vi "HandleObservationSync.vi"(8 "error in (no error)":errorcluster, 11 "S4GUI in":refnum<class "S4GUI.lvclass">) -> (0 "error out":errorcluster, 3 "S4GUI out":refnum<class "S4GUI.lvclass">)   [LabVIEW 2018, in "S4GUI.lvclass"] (continued)
          n221 = call "Read Instrument.lvclass.vi"("error in (no error)"=w570, "S4ACS_GUI in"=w571) -> ("error out"=w541:errorcluster, "Instrument.lvclass"=w542:refnum<class "Instrument.lvclass">, "S4ACS_GUI out"=w572:refnum<class "S4GUI.lvclass">)  [unwired: 7 in]
          n222 = disable-structure shown="Enabled" {
            disable-tunnel: w542 -> [w576 w589]
            disable-tunnel: w541 -> [w575 w588]
            disable-tunnel: [w574 w589] -> w540
            disable-tunnel: [w573 w588] -> w539
            frame Disabled {
              n223 = call "Read WPROT.vi"("error in (no error)"=w575, "Instrument in"=w576) -> ("error out"=w579:errorcluster, "Opt_Selector.lvclass"=w580:refnum<class "Opt_Selector.lvclass">, "Instrument out"=w586:refnum<class "Instrument.lvclass">)  [unwired: 7 in]
              n224 = call-dynamic "Read State Machine.vi"("error in (no error)"=w579, "Device in"=w580) -> ("error out"=w582:errorcluster, "State Machine.lvclass"=w584:refnum<class "State Machine.lvclass">, "Device out"=w581:refnum<class "Opt_Selector.lvclass">)  [unwired: 7 in]
              n225 = call "Next State.vi"("error in (no error)"=w582, "New_State"=30, "State Machine in"=w584) -> ("error out"=w578:errorcluster, "State Machine out"=w577:refnum<class "State Machine.lvclass">)  [unwired: 7 in]
              n226 = call-dynamic "Write State Machine.vi"("error in (no error)"=w578, "State Machine.lvclass"=w577, "Device in"=w581) -> ("error out"=w585:errorcluster, "Device out"=w587:refnum<class "Opt_Selector.lvclass">)  [unwired: 7 in]
              n227 = call "Write WPROT.vi"("error in (no error)"=w585, "Opt_Selector.lvclass"=w587, "Instrument in"=w586) -> ("error out"=w573:errorcluster, "Instrument out"=w574:refnum<class "Instrument.lvclass">)  [unwired: 7 in]
            }
            frame Enabled {
              # "depois do homing no WPSEL, o homing do WPROT é feito automaticamente pelo ICS"
            }
          }
          n228 = call "Read ASEL.vi"("error in (no error)"=w539, "Instrument in"=w540) -> ("error out"=w556:errorcluster, "Opt_Selector.lvclass"=w557:refnum<class "Opt_Selector.lvclass">, "Instrument out"=w563:refnum<class "Instrument.lvclass">)  [unwired: 7 in]
          n229 = call-dynamic "Read State Machine.vi"("error in (no error)"=w556, "Device in"=w557) -> ("error out"=w559:errorcluster, "State Machine.lvclass"=w561:refnum<class "State Machine.lvclass">, "Device out"=w558:refnum<class "Opt_Selector.lvclass">)  [unwired: 7 in]
          n230 = call "Next State.vi"("error in (no error)"=w559, "New_State"=30, "State Machine in"=w561) -> ("error out"=w555:errorcluster, "State Machine out"=w554:refnum<class "State Machine.lvclass">)  [unwired: 7 in]
          n231 = call-dynamic "Write State Machine.vi"("error in (no error)"=w555, "State Machine.lvclass"=w554, "Device in"=w558) -> ("error out"=w562:errorcluster, "Device out"=w564:refnum<class "Opt_Selector.lvclass">)  [unwired: 7 in]
          n232 = Increment(x=w565) -> (x+1=w567:u32)
          n233 = call "Write ASEL.vi"("error in (no error)"=w562, "Opt_Selector.lvclass"=w564, "Instrument in"=w563) -> ("error out"=w537:errorcluster, "Instrument out"=w538:refnum<class "Instrument.lvclass">)  [unwired: 7 in]
          n234 = call "Read GMIR.vi"("error in (no error)"=w537, "Instrument in"=w538) -> ("error out"=w545:errorcluster, "Opt_Continuous.lvclass"=w546:refnum<class "Opt_Continuous.lvclass">, "Instrument out"=w552:refnum<class "Instrument.lvclass">)  [unwired: 7 in]
          n235 = call-dynamic "Read State Machine.vi"("error in (no error)"=w545, "Device in"=w546) -> ("error out"=w548:errorcluster, "State Machine.lvclass"=w550:refnum<class "State Machine.lvclass">, "Device out"=w547:refnum<class "Opt_Continuous.lvclass">)  [unwired: 7 in]
          n236 = call "Next State.vi"("error in (no error)"=w548, "New_State"=30, "State Machine in"=w550) -> ("error out"=w544:errorcluster, "State Machine out"=w543:refnum<class "State Machine.lvclass">)  [unwired: 7 in]
          n237 = call-dynamic "Write State Machine.vi"("error in (no error)"=w544, "State Machine.lvclass"=w543, "Device in"=w547) -> ("error out"=w551:errorcluster, "Device out"=w553:refnum<class "Opt_Continuous.lvclass">)  [unwired: 7 in]
          n238 = call "Write GMIR.vi"("error in (no error)"=w551, "Opt_Continuous.lvclass"=w553, "Instrument in"=w552) -> ("error out"=w536:errorcluster, "Instrument out"=w535:refnum<class "Instrument.lvclass">)  [unwired: 7 in]
          n239 = call "Write Instrument.lvclass.vi"("error in (no error)"=w536, "Instrument.lvclass"=w535, "S4ACS_GUI in"=w572) -> ("error out"=w569:errorcluster, "S4ACS_GUI out"=w568:refnum<class "S4GUI.lvclass">)  [unwired: 7 in]
          n240 = Bundle By Name(cluster=w568, "Obs_state"=w567) -> (w566:refnum<class "S4GUI.lvclass">)
        }
        frame 223 {
          # "Espera terminar o homing de WPROT,ASEL e GFOC\nantes de seguir para o próximo estado."
          n241 = call "Read Instrument.lvclass.vi"("error in (no error)"=w614, "S4ACS_GUI in"=w615) -> ("error out"=w600:errorcluster, "Instrument.lvclass"=w601:refnum<class "Instrument.lvclass">, "S4ACS_GUI out"=w609:refnum<class "S4GUI.lvclass">)  [unwired: 7 in]
          n242 = call "Read ASEL.vi"("error in (no error)"=w600, "Instrument in"=w601) -> ("error out"=w605:errorcluster, "Opt_Selector.lvclass"=w591:refnum<class "Opt_Selector.lvclass">)  [unwired: 7 in, 1 out]
          n243 = call "Read GMIR.vi"("error in (no error)"=w600, "Instrument in"=w601) -> ("error out"=w602:errorcluster, "Opt_Continuous.lvclass"=w590:refnum<class "Opt_Continuous.lvclass">)  [unwired: 7 in, 1 out]
          n244 = disable-structure shown="Enabled" {
            disable-tunnel: [w619 w625] -> w608
            disable-tunnel: w601 -> [w618 _]
            disable-tunnel: w600 -> [w617 w625]
            disable-tunnel: [w616 0 ("State")] -> w599
            frame Disabled {
              n245 = call "Read WPROT.vi"("error in (no error)"=w617, "Instrument in"=w618) -> ("error out"=w621:errorcluster, "Opt_Selector.lvclass"=w620:refnum<class "Opt_Selector.lvclass">)  [unwired: 7 in, 1 out]
              n246 = call-dynamic "Read State Machine.vi"("error in (no error)"=w621, "Device in"=w620) -> ("error out"=w622:errorcluster, "State Machine.lvclass"=w623:refnum<class "State Machine.lvclass">)  [unwired: 7 in, 1 out]
              n247 = call-dynamic "Read State.vi"("error in (no error)"=w622, "State Machine in"=w623) -> ("error out"=w619:errorcluster, "State"=w616:i32)  [unwired: 7 in, 1 out]
            }
            frame Enabled {
            }
          }
          n248 = call-dynamic "Read State Machine.vi"("error in (no error)"=w605, "Device in"=w591) -> ("error out"=w606:errorcluster, "State Machine.lvclass"=w607:refnum<class "State Machine.lvclass">)  [unwired: 7 in, 1 out]
          n249 = call-dynamic "Read State Machine.vi"("error in (no error)"=w602, "Device in"=w590) -> ("error out"=w603:errorcluster, "State Machine.lvclass"=w604:refnum<class "State Machine.lvclass">)  [unwired: 7 in, 1 out]
          n250 = Increment(x=w611) -> (x+1=w610:u32)
          n251 = call-dynamic "Read State.vi"("error in (no error)"=w606, "State Machine in"=w607) -> ("error out"=w594:errorcluster, "State"=w598:i32)  [unwired: 7 in, 1 out]
          n252 = call-dynamic "Read State.vi"("error in (no error)"=w603, "State Machine in"=w604) -> ("error out"=w593:errorcluster, "State"=w597:i32)  [unwired: 7 in, 1 out]
          n253 = Compound Arithmetic op=ADD(w599, w598, w597) -> (w596:i32)
          n254 = Equal To 0?(x=w596) -> (x = 0?=w595:bool)
          n255 = Merge Errors(w608, w594, w593) -> (w592:errorcluster)
          n256 = Select(t=w610, s=w595, f=w611) -> (s? t:f=w612:u32)
          n257 = Bundle By Name(cluster=w609, "Obs_state"=w612) -> (w613:refnum<class "S4GUI.lvclass">)
        }
        frame 224 {
          # "40 x 0.25 = 10s"
          # "40 x 0.25 = 10s"
          # "40 x 0.25 = 10s"
          # "Manda WPSEL para OFF, CALW para OFF e ASEL para OFF"
          n258 = call "Read Instrument.lvclass.vi"("error in (no error)"=w699, "S4ACS_GUI in"=w700) -> ("error out"=w685:errorcluster, "Instrument.lvclass"=w686:refnum<class "Instrument.lvclass">, "S4ACS_GUI out"=w701:refnum<class "S4GUI.lvclass">)  [unwired: 7 in]
          n259 = call "Read WPSEL.vi"("error in (no error)"=w685, "Instrument in"=w686) -> ("error out"=w681:errorcluster, "Opt_Selector.lvclass"=w680:refnum<class "Opt_Selector.lvclass">, "Instrument out"=w693:refnum<class "Instrument.lvclass">)  [unwired: 7 in]
          n260 = call "Write target.vi"("error in (no error)"=w681, "target"=80.0, "Optics in"=w680) -> ("error out"=w684:errorcluster, "Optics out"=w679:refnum<class "Opt_Selector.lvclass">)  [unwired: 7 in]
          n261 = call "Write target name.vi"("error in (no error)"=w684, "target name"="OFF", "Optics in"=w679) -> ("error out"=w677:errorcluster, "Optics out"=w678:refnum<class "Opt_Selector.lvclass">)  [unwired: 7 in]
          n262 = call-dynamic "Read State Machine.vi"("error in (no error)"=w677, "Device in"=w678) -> ("error out"=w688:errorcluster, "State Machine.lvclass"=w690:refnum<class "State Machine.lvclass">, "Device out"=w687:refnum<class "Opt_Selector.lvclass">)  [unwired: 7 in]
          n263 = call "Next State.vi"("error in (no error)"=w688, "New_State"=1, "State Machine in"=w690) -> ("error out"=w638:errorcluster, "State Machine out"=w640:refnum<class "State Machine.lvclass">)  [unwired: 7 in]
          n264 = call-dynamic "Write Timer.vi"("error in (no error)"=w638, "Timer"=u32 40, "State Machine in"=w640) -> ("error out"=w637:errorcluster, "State Machine out"=w639:refnum<class "State Machine.lvclass">)  [unwired: 7 in]
          n265 = call-dynamic "Write State Machine.vi"("error in (no error)"=w637, "State Machine.lvclass"=w639, "Device in"=w687) -> ("error out"=w692:errorcluster, "Device out"=w694:refnum<class "Opt_Selector.lvclass">)  [unwired: 7 in]
          n266 = Increment(x=w691) -> (x+1=w696:u32)
          n267 = call "Write WPSEL.vi"("error in (no error)"=w692, "Opt_Selector.lvclass"=w694, "Instrument in"=w693) -> ("error out"=w652:errorcluster, "Instrument out"=w651:refnum<class "Instrument.lvclass">)  [unwired: 7 in]
          n268 = call "Read CALW.vi"("error in (no error)"=w652, "Instrument in"=w651) -> ("error out"=w668:errorcluster, "Opt_Selector.lvclass"=w650:refnum<class "Opt_Selector.lvclass">, "Instrument out"=w648:refnum<class "Instrument.lvclass">)  [unwired: 7 in]
          n269 = call "Write target.vi"("error in (no error)"=w668, "target"=0.0, "Optics in"=w650) -> ("error out"=w671:errorcluster, "Optics out"=w667:refnum<class "Opt_Selector.lvclass">)  [unwired: 7 in]
          n270 = call "Write target name.vi"("error in (no error)"=w671, "target name"="OFF", "Optics in"=w667) -> ("error out"=w665:errorcluster, "Optics out"=w666:refnum<class "Opt_Selector.lvclass">)  [unwired: 7 in]
          n271 = call-dynamic "Read State Machine.vi"("error in (no error)"=w665, "Device in"=w666) -> ("error out"=w673:errorcluster, "State Machine.lvclass"=w675:refnum<class "State Machine.lvclass">, "Device out"=w672:refnum<class "Opt_Selector.lvclass">)  [unwired: 7 in]
          n272 = call "Next State.vi"("error in (no error)"=w673, "New_State"=1, "State Machine in"=w675) -> ("error out"=w634:errorcluster, "State Machine out"=w635:refnum<class "State Machine.lvclass">)  [unwired: 7 in]
          n273 = call-dynamic "Write Timer.vi"("error in (no error)"=w634, "Timer"=u32 40, "State Machine in"=w635) -> ("error out"=w633:errorcluster, "State Machine out"=w632:refnum<class "State Machine.lvclass">)  [unwired: 7 in]
          n274 = call-dynamic "Write State Machine.vi"("error in (no error)"=w633, "State Machine.lvclass"=w632, "Device in"=w672) -> ("error out"=w676:errorcluster, "Device out"=w649:refnum<class "Opt_Selector.lvclass">)  [unwired: 7 in]
          n275 = call "Write CALW.vi"("error in (no error)"=w676, "Opt_Selector.lvclass"=w649, "Instrument in"=w648) -> ("error out"=w647:errorcluster, "Instrument out"=w646:refnum<class "Instrument.lvclass">)  [unwired: 7 in]
          n276 = call "Read ASEL.vi"("error in (no error)"=w647, "Instrument in"=w646) -> ("error out"=w656:errorcluster, "Opt_Selector.lvclass"=w645:refnum<class "Opt_Selector.lvclass">, "Instrument out"=w643:refnum<class "Instrument.lvclass">)  [unwired: 7 in]
          n277 = call "Write target.vi"("error in (no error)"=w656, "target"=0.0, "Optics in"=w645) -> ("error out"=w659:errorcluster, "Optics out"=w655:refnum<class "Opt_Selector.lvclass">)  [unwired: 7 in]
          n278 = call "Write target name.vi"("error in (no error)"=w659, "target name"="OFF", "Optics in"=w655) -> ("error out"=w653:errorcluster, "Optics out"=w654:refnum<class "Opt_Selector.lvclass">)  [unwired: 7 in]
          n279 = call-dynamic "Read State Machine.vi"("error in (no error)"=w653, "Device in"=w654) -> ("error out"=w661:errorcluster, "State Machine.lvclass"=w663:refnum<class "State Machine.lvclass">, "Device out"=w660:refnum<class "Opt_Selector.lvclass">)  [unwired: 7 in]
          n280 = call "Next State.vi"("error in (no error)"=w661, "New_State"=1, "State Machine in"=w663) -> ("error out"=w628:errorcluster, "State Machine out"=w629:refnum<class "State Machine.lvclass">)  [unwired: 7 in]
          n281 = call-dynamic "Write Timer.vi"("error in (no error)"=w628, "Timer"=u32 40, "State Machine in"=w629) -> ("error out"=w627:errorcluster, "State Machine out"=w626:refnum<class "State Machine.lvclass">)  [unwired: 7 in]
          n282 = call-dynamic "Write State Machine.vi"("error in (no error)"=w627, "State Machine.lvclass"=w626, "Device in"=w660) -> ("error out"=w664:errorcluster, "Device out"=w644:refnum<class "Opt_Selector.lvclass">)  [unwired: 7 in]
          n283 = call "Write ASEL.vi"("error in (no error)"=w664, "Opt_Selector.lvclass"=w644, "Instrument in"=w643) -> ("error out"=w641:errorcluster, "Instrument out"=w642:refnum<class "Instrument.lvclass">)  [unwired: 7 in]
          n284 = call "Write Instrument.lvclass.vi"("error in (no error)"=w641, "Instrument.lvclass"=w642, "S4ACS_GUI in"=w701) -> ("error out"=w698:errorcluster, "S4ACS_GUI out"=w697:refnum<class "S4GUI.lvclass">)  [unwired: 7 in]
          n285 = Bundle By Name(cluster=w697, "Obs_state"=w696) -> (w695:refnum<class "S4GUI.lvclass">)
        }
        frame 225 {
          # "Espera terminar o movimento de WPSEL, ASEL e CALW para CLEAR."
          n286 = call "Read Instrument.lvclass.vi"("error in (no error)"=w730, "S4ACS_GUI in"=w731) -> ("error out"=w713:errorcluster, "Instrument.lvclass"=w714:refnum<class "Instrument.lvclass">, "S4ACS_GUI out"=w722:refnum<class "S4GUI.lvclass">)  [unwired: 7 in]
          n287 = call "Read ASEL.vi"("error in (no error)"=w713, "Instrument in"=w714) -> ("error out"=w718:errorcluster, "Opt_Selector.lvclass"=w704:refnum<class "Opt_Selector.lvclass">)  [unwired: 7 in, 1 out]
          n288 = call "Read CALW.vi"("error in (no error)"=w713, "Instrument in"=w714) -> ("error out"=w715:errorcluster, "Opt_Selector.lvclass"=w703:refnum<class "Opt_Selector.lvclass">)  [unwired: 7 in, 1 out]
          n289 = call "Read WPSEL.vi"("error in (no error)"=w713, "Instrument in"=w714) -> ("error out"=w727:errorcluster, "Opt_Selector.lvclass"=w726:refnum<class "Opt_Selector.lvclass">)  [unwired: 7 in, 1 out]
          n290 = call-dynamic "Read State Machine.vi"("error in (no error)"=w715, "Device in"=w703) -> ("error out"=w716:errorcluster, "State Machine.lvclass"=w717:refnum<class "State Machine.lvclass">)  [unwired: 7 in, 1 out]
          n291 = call-dynamic "Read State Machine.vi"("error in (no error)"=w718, "Device in"=w704) -> ("error out"=w719:errorcluster, "State Machine.lvclass"=w720:refnum<class "State Machine.lvclass">)  [unwired: 7 in, 1 out]
          n292 = call-dynamic "Read State Machine.vi"("error in (no error)"=w727, "Device in"=w726) -> ("error out"=w728:errorcluster, "State Machine.lvclass"=w729:refnum<class "State Machine.lvclass">)  [unwired: 7 in, 1 out]
          n293 = call-dynamic "Read State.vi"("error in (no error)"=w719, "State Machine in"=w720) -> ("error out"=w707:errorcluster, "State"=w711:i32)  [unwired: 7 in, 1 out]
          n294 = call-dynamic "Read State.vi"("error in (no error)"=w716, "State Machine in"=w717) -> ("error out"=w706:errorcluster, "State"=w710:i32)  [unwired: 7 in, 1 out]
          n295 = call-dynamic "Read State.vi"("error in (no error)"=w728, "State Machine in"=w729) -> ("error out"=w721:errorcluster, "State"=w712:i32)  [unwired: 7 in, 1 out]
          n296 = Compound Arithmetic op=ADD(w712, w711, w710) -> (w709:i32)
          n297 = Equal To 0?(x=w709) -> (x = 0?=w708:bool)
          n298 = Merge Errors(w721, w707, w706) -> (w705:errorcluster)
          n299 = Select(t=u32 0, s=w708, f=w723) -> (s? t:f=w724:u32)
          n300 = Bundle By Name(cluster=w722, "Obs_state"=w724) -> (w725:refnum<class "S4GUI.lvclass">)
        }
        frame 230 {
          # "PARK:\nWPSEL = OFF\n(WPROT=NA)\nCALW=SHUTTER\nASEL=OFF"
          n301 = call "Read Instrument.lvclass.vi"("error in (no error)"=w800, "S4ACS_GUI in"=w801) -> ("error out"=w793:errorcluster, "Instrument.lvclass"=w794:refnum<class "Instrument.lvclass">, "S4ACS_GUI out"=w735:refnum<class "S4GUI.lvclass">)  [unwired: 7 in]
          n302 = call "Read WPSEL.vi"("error in (no error)"=w793, "Instrument in"=w794) -> ("error out"=w756:errorcluster, "Opt_Selector.lvclass"=w759:refnum<class "Opt_Selector.lvclass">, "Instrument out"=w789:refnum<class "Instrument.lvclass">)  [unwired: 7 in]
          n303 = call "Write target name.vi"("error in (no error)"=w756, "target name"="OFF", "Optics in"=w759) -> ("error out"=w755:errorcluster, "Optics out"=w758:refnum<class "Opt_Selector.lvclass">)  [unwired: 7 in]
          n304 = call "Write target.vi"("error in (no error)"=w755, "target"=80.0, "Optics in"=w758) -> ("error out"=w754:errorcluster, "Optics out"=w757:refnum<class "Opt_Selector.lvclass">)  [unwired: 7 in]
          n305 = call-dynamic "Read State Machine.vi"("error in (no error)"=w754, "Device in"=w757) -> ("error out"=w785:errorcluster, "State Machine.lvclass"=w787:refnum<class "State Machine.lvclass">, "Device out"=w784:refnum<class "Opt_Selector.lvclass">)  [unwired: 7 in]
          n306 = call "Next State.vi"("error in (no error)"=w785, "New_State"=1, "State Machine in"=w787) -> ("error out"=w764:errorcluster, "State Machine out"=w765:refnum<class "State Machine.lvclass">)  [unwired: 7 in]
          n307 = call-dynamic "Write State Machine.vi"("error in (no error)"=w764, "State Machine.lvclass"=w765, "Device in"=w784) -> ("error out"=w788:errorcluster, "Device out"=w790:refnum<class "Opt_Selector.lvclass">)  [unwired: 7 in]
          n308 = Increment(x=w795) -> (x+1=w797:u32)
          n309 = call "Write WPSEL.vi"("error in (no error)"=w788, "Opt_Selector.lvclass"=w790, "Instrument in"=w789) -> ("error out"=w768:errorcluster, "Instrument out"=w769:refnum<class "Instrument.lvclass">)  [unwired: 7 in]
          n310 = call "Read CALW.vi"("error in (no error)"=w768, "Instrument in"=w769) -> ("error out"=w748:errorcluster, "Opt_Selector.lvclass"=w747:refnum<class "Opt_Selector.lvclass">, "Instrument out"=w782:refnum<class "Instrument.lvclass">)  [unwired: 7 in]
          n311 = call "Write target name.vi"("error in (no error)"=w748, "target name"="SHUTTER", "Optics in"=w747) -> ("error out"=w751:errorcluster, "Optics out"=w746:refnum<class "Opt_Selector.lvclass">)  [unwired: 7 in]
          n312 = call "Write target.vi"("error in (no error)"=w751, "target"=216.0, "Optics in"=w746) -> ("error out"=w744:errorcluster, "Optics out"=w745:refnum<class "Opt_Selector.lvclass">)  [unwired: 7 in]
          n313 = call-dynamic "Read State Machine.vi"("error in (no error)"=w744, "Device in"=w745) -> ("error out"=w778:errorcluster, "State Machine.lvclass"=w780:refnum<class "State Machine.lvclass">, "Device out"=w777:refnum<class "Opt_Selector.lvclass">)  [unwired: 7 in]
          n314 = call "Next State.vi"("error in (no error)"=w778, "New_State"=1, "State Machine in"=w780) -> ("error out"=w762:errorcluster, "State Machine out"=w763:refnum<class "State Machine.lvclass">)  [unwired: 7 in]
          n315 = call-dynamic "Write State Machine.vi"("error in (no error)"=w762, "State Machine.lvclass"=w763, "Device in"=w777) -> ("error out"=w781:errorcluster, "Device out"=w783:refnum<class "Opt_Selector.lvclass">)  [unwired: 7 in]
          n316 = call "Write CALW.vi"("error in (no error)"=w781, "Opt_Selector.lvclass"=w783, "Instrument in"=w782) -> ("error out"=w766:errorcluster, "Instrument out"=w767:refnum<class "Instrument.lvclass">)  [unwired: 7 in]
          n317 = call "Read ASEL.vi"("error in (no error)"=w766, "Instrument in"=w767) -> ("error out"=w737:errorcluster, "Opt_Selector.lvclass"=w740:refnum<class "Opt_Selector.lvclass">, "Instrument out"=w775:refnum<class "Instrument.lvclass">)  [unwired: 7 in]
          n318 = call "Write target name.vi"("error in (no error)"=w737, "target name"="OFF", "Optics in"=w740) -> ("error out"=w743:errorcluster, "Optics out"=w739:refnum<class "Opt_Selector.lvclass">)  [unwired: 7 in]
          n319 = call "Write target.vi"("error in (no error)"=w743, "target"=0.0, "Optics in"=w739) -> ("error out"=w736:errorcluster, "Optics out"=w738:refnum<class "Opt_Selector.lvclass">)  [unwired: 7 in]
          n320 = call-dynamic "Read State Machine.vi"("error in (no error)"=w736, "Device in"=w738) -> ("error out"=w771:errorcluster, "State Machine.lvclass"=w773:refnum<class "State Machine.lvclass">, "Device out"=w770:refnum<class "Opt_Selector.lvclass">)  [unwired: 7 in]
          n321 = call "Next State.vi"("error in (no error)"=w771, "New_State"=1, "State Machine in"=w773) -> ("error out"=w760:errorcluster, "State Machine out"=w761:refnum<class "State Machine.lvclass">)  [unwired: 7 in]
          n322 = call-dynamic "Write State Machine.vi"("error in (no error)"=w760, "State Machine.lvclass"=w761, "Device in"=w770) -> ("error out"=w774:errorcluster, "Device out"=w776:refnum<class "Opt_Selector.lvclass">)  [unwired: 7 in]
          n323 = call "Write ASEL.vi"("error in (no error)"=w774, "Opt_Selector.lvclass"=w776, "Instrument in"=w775) -> ("error out"=w792:errorcluster, "Instrument out"=w791:refnum<class "Instrument.lvclass">)  [unwired: 7 in]
          n324 = Tick Count (ms)() -> (millisecond timer value=w732:u32)
          n325 = local write "time1"(w732) -> ()
          n326 = Bundle By Name(cluster=w735, "Error Msg"="Parking in progress. Wait....") -> (w734:refnum<class "S4GUI.lvclass">)
          n327 = call "Write Instrument.lvclass.vi"("error in (no error)"=w792, "Instrument.lvclass"=w791, "S4ACS_GUI in"=w734) -> ("error out"=w799:errorcluster, "S4ACS_GUI out"=w798:refnum<class "S4GUI.lvclass">)  [unwired: 7 in]
          n328 = Bundle By Name(cluster=w798, "Obs_state"=w797) -> (w796:refnum<class "S4GUI.lvclass">)
        }
        frame 231 {
          # "Espera terminar o parking de WPSEL,CALW e ASEL\nantes de encerrar aplicacao (exit=True)."
          n329 = call "Read Instrument.lvclass.vi"("error in (no error)"=w837, "S4ACS_GUI in"=w838) -> ("error out"=w821:errorcluster, "Instrument.lvclass"=w822:refnum<class "Instrument.lvclass">, "S4ACS_GUI out"=w830:refnum<class "S4GUI.lvclass">)  [unwired: 7 in]
          n330 = call "Read CALW.vi"("error in (no error)"=w821, "Instrument in"=w822) -> ("error out"=w826:errorcluster, "Opt_Selector.lvclass"=w812:refnum<class "Opt_Selector.lvclass">)  [unwired: 7 in, 1 out]
          n331 = call "Read ASEL.vi"("error in (no error)"=w821, "Instrument in"=w822) -> ("error out"=w823:errorcluster, "Opt_Selector.lvclass"=w811:refnum<class "Opt_Selector.lvclass">)  [unwired: 7 in, 1 out]
          n332 = call "Read WPSEL.vi"("error in (no error)"=w821, "Instrument in"=w822) -> ("error out"=w834:errorcluster, "Opt_Selector.lvclass"=w833:refnum<class "Opt_Selector.lvclass">)  [unwired: 7 in, 1 out]
          n333 = call-dynamic "Read State Machine.vi"("error in (no error)"=w826, "Device in"=w812) -> ("error out"=w827:errorcluster, "State Machine.lvclass"=w828:refnum<class "State Machine.lvclass">)  [unwired: 7 in, 1 out]
          n334 = call-dynamic "Read State Machine.vi"("error in (no error)"=w823, "Device in"=w811) -> ("error out"=w824:errorcluster, "State Machine.lvclass"=w825:refnum<class "State Machine.lvclass">)  [unwired: 7 in, 1 out]
          n335 = call-dynamic "Read State Machine.vi"("error in (no error)"=w834, "Device in"=w833) -> ("error out"=w835:errorcluster, "State Machine.lvclass"=w836:refnum<class "State Machine.lvclass">)  [unwired: 7 in, 1 out]
          n336 = Increment(x=w804) -> (x+1=w831:u32)
          n337 = call-dynamic "Read State.vi"("error in (no error)"=w827, "State Machine in"=w828) -> ("error out"=w815:errorcluster, "State"=w819:i32)  [unwired: 7 in, 1 out]
          n338 = call-dynamic "Read State.vi"("error in (no error)"=w824, "State Machine in"=w825) -> ("error out"=w814:errorcluster, "State"=w818:i32)  [unwired: 7 in, 1 out]
          n339 = call-dynamic "Read State.vi"("error in (no error)"=w835, "State Machine in"=w836) -> ("error out"=w829:errorcluster, "State"=w820:i32)  [unwired: 7 in, 1 out]
          n340 = Compound Arithmetic op=ADD(w820, w819, w818) -> (w817:i32)
          n341 = Equal To 0?(x=w817) -> (x = 0?=w816:bool)
          n342 = Merge Errors(w829, w815, w814) -> (w813:errorcluster)
          n343 = Select(t=w831, s=w816, f=w804) -> (s? t:f=w803:u32)
          n344 = Tick Count (ms)() -> (millisecond timer value=w810:u32)
          n345 = local read "time1"() -> (w808:u32)
          n346 = Subtract(x=w810, y=w808) -> (x-y=w809:u32)
          n347 = To Double Precision Float(number=w809) -> (double precision float=w807:dbl)
          n348 = Greater?(x=w807, y=30000.0) -> (0:w805:bool)
          n349 = case shown="True" w805 {
            tunnel: w804 -> [_ w841]
            tunnel: [w839 w840] -> w802
            tunnel: w803 -> [w839 _]
            frame False {
            }
            frame True {
              n350 = Increment(x=w841) -> (x+1=w840:u32)
            }
          }
          n351 = Bundle By Name(cluster=w830, "Obs_state"=w802) -> (w832:refnum<class "S4GUI.lvclass">)
        }
        frame 232 {
          n352 = Increment(x=w843) -> (x+1=w842:u32)
          n353 = Tick Count (ms)() -> (millisecond timer value=w844:u32)
          n354 = local write "time1"(w844) -> ()
          n355 = Bundle By Name(cluster=w847, "Obs_state"=w842) -> (w845:refnum<class "S4GUI.lvclass">)
        }
        frame 233 {
          # "Aguarda 1s para atualização do painel da GUI antes de encerrar..."
          n356 = local read "time1"() -> (w851:u32)
          n357 = Tick Count (ms)() -> (millisecond timer value=w852:u32)
          n358 = Subtract(x=w852, y=w851) -> (x-y=w850:u32)
          n359 = Greater?(x=w850, y=u32 1000) -> (0:w848:bool)
          n360 = case shown="True" w848 {
            tunnel: w854 -> [w858 w860]
            tunnel: [w858 w859] -> w853
            frame False {
            }
            frame True {
              n361 = Increment(x=w860) -> (x+1=w859:u32)
            }
          }
          n362 = Bundle By Name(cluster=w857, "Obs_state"=w853) -> (w855:refnum<class "S4GUI.lvclass">)
        }
        frame 234 {
          n363 = Bundle By Name(cluster=w865, "Obs_state"=u32 0, "exit"=TRUE) -> (w863:refnum<class "S4GUI.lvclass">)
        }
        frame 240 {
          # "Carrega mensagem de \"Invalid temperature\" (botão SET da aba \"CCD temp\" de cada canal) e desvia para estado de erro (Obs_state=1)"
          n364 = Bundle By Name(cluster=w869, "Error Msg"="ERROR Invalid temperature - input value lower than minimum for current CCD setup (state 240). " ("f"), "Obs_state"=u32 1) -> (w868:refnum<class "S4GUI.lvclass">)
        }
        frame 251 {
          # "Verifica se ha funcao valida de instrumento:"
          n365 = flat-sequence {
            tunnel: w882 -> [w1092]
            tunnel: [w1092] -> w873
            frame #0 {
              n366 = Tick Count (ms)() -> (millisecond timer value=→"time3":u32)
            }
          }
          n367 = Unbundle By Name(w879) -> ("Instrument.lvclass"=w876:refnum<class "Instrument.lvclass">)
          n368 = call-dynamic "Load Function.vi"("error in (no error)"=w873, "Instrument in"=w876) -> ("error out"=w872:errorcluster, "Instrument out"=w875:refnum<class "Instrument.lvclass">)  [unwired: 8 in]
          n369 = call-dynamic "Read Function.vi"("error in (no error)"=w872, "Instrument in"=w875) -> ("error out"=w871:errorcluster, "Function"=w877:enum16{"PHOTO", "POLAR", "NONE"}, "Instrument out"=w874:refnum<class "Instrument.lvclass">)  [unwired: 7 in]
          n370 = Bundle By Name(cluster=w879, "Instrument.lvclass"=w874) -> (w878:refnum<class "S4GUI.lvclass">)
          n371 = case shown="Default" w877 {
            tunnel: w878 -> [w891 w954]
            tunnel: w886 -> [_ w951]
            tunnel: [u32 1 ("Obs_state") w950] -> w885
            tunnel: [w890 w940] -> w884
            tunnel: [w891 w939] -> w883
            tunnel: w871 -> [w890 w938]
            tunnel: ["ERROR: No instrument function set (neither POLARIMETRICS nor PHOTOMETRICS )" ("Error Msg") w916] -> w880
            frame "NONE" {
              # "Nenhuma função valida: nem polarimetria nem fotometria..."
            }
            frame Default {
              # "POLAR ou PHOTO"
              n372 = call-dynamic "Read AcquisitionA.vi"("error in (no error)"=w938, "S4ACS_GUI in"=w954) -> ("error out"=w924:errorcluster, "Acquisition.lvclass"=w922:refnum<class "Acquisition.lvclass">, "S4ACS_GUI out"=w956:refnum<class "S4GUI.lvclass">)  [unwired: 7 in]
              n373 = call-dynamic "Read enabled.vi"("error in (no error)"=w924, "Server in"=w922) -> ("error out"=w923:errorcluster, "enabled"=w919:bool, "Server out"=w921:refnum<class "Acquisition.lvclass">)  [unwired: 7 in]
              n374 = call "Read connection.vi"("error in (no error)"=w923, "Server in"=w921) -> ("error out"=w953:errorcluster, "connection"=w925:bool, "Server out"=w952:refnum<class "Acquisition.lvclass">)  [unwired: 7 in]
              n375 = And(x=w925, y=w919) -> (x .and. y?=w920:bool)
              n376 = case shown="False" w920 {
                tunnel: [w1072 w1091] -> w957
                tunnel: [w1071 w1090] -> w955
                tunnel: w953 -> [w1071 w1089]
                tunnel: w952 -> [w1072 w1088]
                tunnel: w919 -> [w1068 _]
                tunnel: [w1067 u32 0] -> w918
                frame False {
                  n377 = Select(t=u32 1, s=w1068, f=u32 0) -> (s? t:f=w1067:u32)
                }
                frame True {
                  # "configura o canal,\nmas não dispara\na exposicao."
                  n378 = call-dynamic "Read Channel.vi"("error in (no error)"=w1089, "Acquisition in"=w1088) -> ("error out"=w1078:errorcluster, "Channel.lvclass"=w1080:refnum<class "Channel.lvclass">, "Acquisition out"=w1087:refnum<class "Acquisition.lvclass">)  [unwired: 7 in]
                  n379 = call-dynamic "Write expose.vi"("error in (no error)"=w1078, "expose"=FALSE, "Channel in"=w1080) -> ("error out"=w1077:errorcluster, "Channel out"=w1079:refnum<class "Channel.lvclass">)  [unwired: 7 in]
                  n380 = call-dynamic "Read State Machine.vi"("error in (no error)"=w1077, "Device in"=w1079) -> ("error out"=w1084:errorcluster, "State Machine.lvclass"=w1086:refnum<class "State Machine.lvclass">, "Device out"=w1082:refnum<class "Channel.lvclass">)  [unwired: 7 in]
                  n381 = call "Next State.vi"("error in (no error)"=w1084, "New_State"=1, "State Machine in"=w1086) -> ("error out"=w1074:errorcluster, "State Machine out"=w1075:refnum<class "State Machine.lvclass">)  [unwired: 7 in]
                  n382 = call-dynamic "Write State Machine.vi"("error in (no error)"=w1074, "State Machine.lvclass"=w1075, "Device in"=w1082) -> ("error out"=w1081:errorcluster, "Device out"=w1083:refnum<class "Channel.lvclass">)  [unwired: 7 in]
                  n383 = call-dynamic "Write Channel.vi"("error in (no error)"=w1081, "Channel.lvclass"=w1083, "Acquisition in"=w1087) -> ("error out"=w1090:errorcluster, "Acquisition out"=w1091:refnum<class "Acquisition.lvclass">)  [unwired: 7 in]
                }
              }
              n384 = call-dynamic "Write AcquisitionA.vi"("error in (no error)"=w955, "Acquisition.lvclass"=w957, "S4ACS_GUI in"=w956) -> ("error out"=w948:errorcluster, "S4ACS_GUI out"=w947:refnum<class "S4GUI.lvclass">)  [unwired: 7 in]
              n385 = call "Read AcquisitionB.vi"("error in (no error)"=w948, "S4ACS_GUI in"=w947) -> ("error out"=w908:errorcluster, "Acquisition.lvclass"=w910:refnum<class "Acquisition.lvclass">, "S4ACS_GUI out"=w949:refnum<class "S4GUI.lvclass">)  [unwired: 7 in]
              n386 = call-dynamic "Read enabled.vi"("error in (no error)"=w908, "Server in"=w910) -> ("error out"=w907:errorcluster, "enabled"=w892:bool, "Server out"=w909:refnum<class "Acquisition.lvclass">)  [unwired: 7 in]
              n387 = call "Read connection.vi"("error in (no error)"=w907, "Server in"=w909) -> ("error out"=w936:errorcluster, "connection"=w911:bool, "Server out"=w937:refnum<class "Acquisition.lvclass">)  [unwired: 7 in]
              n388 = And(x=w911, y=w892) -> (x .and. y?=w912:bool)
              n389 = case shown="False" w912 {
                tunnel: [w1047 w1066] -> w935
                tunnel: [w1046 w1065] -> w934
                tunnel: w936 -> [w1046 w1064]
                tunnel: w937 -> [w1047 w1063]
                tunnel: [w1043 u32 0 ("f")] -> w915
                tunnel: w892 -> [w1042 _]
                frame False {
                  n390 = Select(t=u32 2, s=w1042, f=u32 0) -> (s? t:f=w1043:u32)
                }
                frame True {
                  # "configura o canal,\nmas não dispara\na exposicao."
                  n391 = call-dynamic "Read Channel.vi"("error in (no error)"=w1064, "Acquisition in"=w1063) -> ("error out"=w1053:errorcluster, "Channel.lvclass"=w1055:refnum<class "Channel.lvclass">, "Acquisition out"=w1062:refnum<class "Acquisition.lvclass">)  [unwired: 7 in]
                  n392 = call-dynamic "Write expose.vi"("error in (no error)"=w1053, "expose"=FALSE, "Channel in"=w1055) -> ("error out"=w1052:errorcluster, "Channel out"=w1054:refnum<class "Channel.lvclass">)  [unwired: 7 in]
                  n393 = call-dynamic "Read State Machine.vi"("error in (no error)"=w1052, "Device in"=w1054) -> ("error out"=w1059:errorcluster, "State Machine.lvclass"=w1061:refnum<class "State Machine.lvclass">, "Device out"=w1057:refnum<class "Channel.lvclass">)  [unwired: 7 in]
                  n394 = call "Next State.vi"("error in (no error)"=w1059, "New_State"=1, "State Machine in"=w1061) -> ("error out"=w1049:errorcluster, "State Machine out"=w1050:refnum<class "State Machine.lvclass">)  [unwired: 7 in]
                  n395 = call-dynamic "Write State Machine.vi"("error in (no error)"=w1049, "State Machine.lvclass"=w1050, "Device in"=w1057) -> ("error out"=w1056:errorcluster, "Device out"=w1058:refnum<class "Channel.lvclass">)  [unwired: 7 in]
                  n396 = call-dynamic "Write Channel.vi"("error in (no error)"=w1056, "Channel.lvclass"=w1058, "Acquisition in"=w1062) -> ("error out"=w1065:errorcluster, "Acquisition out"=w1066:refnum<class "Acquisition.lvclass">)  [unwired: 7 in]
                }
              }
              n397 = call "Write AcquisitionB.vi"("error in (no error)"=w934, "Acquisition.lvclass"=w935, "S4ACS_GUI in"=w949) -> ("error out"=w944:errorcluster, "S4ACS_GUI out"=w943:refnum<class "S4GUI.lvclass">)  [unwired: 7 in]
              n398 = call-dynamic "Read AcquisitionC.vi"("error in (no error)"=w944, "S4ACS_GUI in"=w943) -> ("error out"=w904:errorcluster, "Acquisition.lvclass"=w906:refnum<class "Acquisition.lvclass">, "S4ACS_GUI out"=w946:refnum<class "S4GUI.lvclass">)  [unwired: 7 in]
              n399 = call-dynamic "Read enabled.vi"("error in (no error)"=w904, "Server in"=w906) -> ("error out"=w903:errorcluster, "enabled"=w893:bool, "Server out"=w905:refnum<class "Acquisition.lvclass">)  [unwired: 7 in]
              n400 = call "Read connection.vi"("error in (no error)"=w903, "Server in"=w905) -> ("error out"=w932:errorcluster, "connection"=w902:bool, "Server out"=w933:refnum<class "Acquisition.lvclass">)  [unwired: 7 in]
              n401 = And(x=w902, y=w893) -> (x .and. y?=w901:bool)
              n402 = case shown="True" w901 {
                tunnel: [w1022 w1041] -> w931
                tunnel: [w1021 w1040] -> w930
                tunnel: w932 -> [w1021 w1039]
                tunnel: w933 -> [w1022 w1038]
                tunnel: [w1018 u32 0 ("f")] -> w914
                tunnel: w893 -> [w1017 _]
                frame False {
                  n403 = Select(t=u32 4, s=w1017, f=u32 0) -> (s? t:f=w1018:u32)
                }
                frame True {
                  # "configura o canal,\nmas não dispara\na exposicao."
                  n404 = call-dynamic "Read Channel.vi"("error in (no error)"=w1039, "Acquisition in"=w1038) -> ("error out"=w1028:errorcluster, "Channel.lvclass"=w1030:refnum<class "Channel.lvclass">, "Acquisition out"=w1037:refnum<class "Acquisition.lvclass">)  [unwired: 7 in]
                  n405 = call-dynamic "Write expose.vi"("error in (no error)"=w1028, "expose"=FALSE, "Channel in"=w1030) -> ("error out"=w1027:errorcluster, "Channel out"=w1029:refnum<class "Channel.lvclass">)  [unwired: 7 in]
                  n406 = call-dynamic "Read State Machine.vi"("error in (no error)"=w1027, "Device in"=w1029) -> ("error out"=w1034:errorcluster, "State Machine.lvclass"=w1036:refnum<class "State Machine.lvclass">, "Device out"=w1032:refnum<class "Channel.lvclass">)  [unwired: 7 in]
                  n407 = call "Next State.vi"("error in (no error)"=w1034, "New_State"=1, "State Machine in"=w1036) -> ("error out"=w1024:errorcluster, "State Machine out"=w1025:refnum<class "State Machine.lvclass">)  [unwired: 7 in]
                  n408 = call-dynamic "Write State Machine.vi"("error in (no error)"=w1024, "State Machine.lvclass"=w1025, "Device in"=w1032) -> ("error out"=w1031:errorcluster, "Device out"=w1033:refnum<class "Channel.lvclass">)  [unwired: 7 in]
                  n409 = call-dynamic "Write Channel.vi"("error in (no error)"=w1031, "Channel.lvclass"=w1033, "Acquisition in"=w1037) -> ("error out"=w1040:errorcluster, "Acquisition out"=w1041:refnum<class "Acquisition.lvclass">)  [unwired: 7 in]
                }
              }
              n410 = call-dynamic "Write AcquisitionC.vi"("error in (no error)"=w930, "Acquisition.lvclass"=w931, "S4ACS_GUI in"=w946) -> ("error out"=w942:errorcluster, "S4ACS_GUI out"=w941:refnum<class "S4GUI.lvclass">)  [unwired: 7 in]
              n411 = call-dynamic "Read AcquisitionD.vi"("error in (no error)"=w942, "S4ACS_GUI in"=w941) -> ("error out"=w898:errorcluster, "Acquisition.lvclass"=w900:refnum<class "Acquisition.lvclass">, "S4ACS_GUI out"=w945:refnum<class "S4GUI.lvclass">)  [unwired: 7 in]
              n412 = call-dynamic "Read enabled.vi"("error in (no error)"=w898, "Server in"=w900) -> ("error out"=w897:errorcluster, "enabled"=w894:bool, "Server out"=w899:refnum<class "Acquisition.lvclass">)  [unwired: 7 in]
              n413 = call "Read connection.vi"("error in (no error)"=w897, "Server in"=w899) -> ("error out"=w928:errorcluster, "connection"=w896:bool, "Server out"=w929:refnum<class "Acquisition.lvclass">)  [unwired: 7 in]
              n414 = And(x=w896, y=w894) -> (x .and. y?=w895:bool)
              n415 = case shown="True" w895 {
                tunnel: [w997 w1016] -> w927
                tunnel: [w996 w1015] -> w926
                tunnel: w928 -> [w996 w1014]
                tunnel: w929 -> [w997 w1013]
                tunnel: [w993 u32 0 ("f")] -> w913
                tunnel: w894 -> [w992 _]
                frame False {
                  n416 = Select(t=u32 8, s=w992, f=u32 0) -> (s? t:f=w993:u32)
                }
                frame True {
                  # "configura o canal,\nmas não dispara\na exposicao."
                  n417 = call-dynamic "Read Channel.vi"("error in (no error)"=w1014, "Acquisition in"=w1013) -> ("error out"=w1003:errorcluster, "Channel.lvclass"=w1005:refnum<class "Channel.lvclass">, "Acquisition out"=w1012:refnum<class "Acquisition.lvclass">)  [unwired: 7 in]
                  n418 = call-dynamic "Write expose.vi"("error in (no error)"=w1003, "expose"=FALSE, "Channel in"=w1005) -> ("error out"=w1002:errorcluster, "Channel out"=w1004:refnum<class "Channel.lvclass">)  [unwired: 7 in]
                  n419 = call-dynamic "Read State Machine.vi"("error in (no error)"=w1002, "Device in"=w1004) -> ("error out"=w1009:errorcluster, "State Machine.lvclass"=w1011:refnum<class "State Machine.lvclass">, "Device out"=w1007:refnum<class "Channel.lvclass">)  [unwired: 7 in]
                  n420 = call "Next State.vi"("error in (no error)"=w1009, "New_State"=1, "State Machine in"=w1011) -> ("error out"=w999:errorcluster, "State Machine out"=w1000:refnum<class "State Machine.lvclass">)  [unwired: 7 in]
                  n421 = call-dynamic "Write State Machine.vi"("error in (no error)"=w999, "State Machine.lvclass"=w1000, "Device in"=w1007) -> ("error out"=w1006:errorcluster, "Device out"=w1008:refnum<class "Channel.lvclass">)  [unwired: 7 in]
                  n422 = call-dynamic "Write Channel.vi"("error in (no error)"=w1006, "Channel.lvclass"=w1008, "Acquisition in"=w1012) -> ("error out"=w1015:errorcluster, "Acquisition out"=w1016:refnum<class "Acquisition.lvclass">)  [unwired: 7 in]
                }
              }
              n423 = call-dynamic "Write AcquisitionD.vi"("error in (no error)"=w926, "Acquisition.lvclass"=w927, "S4ACS_GUI in"=w945) -> ("error out"=w940:errorcluster, "S4ACS_GUI out"=w939:refnum<class "S4GUI.lvclass">)  [unwired: 7 in]
              n424 = Compound Arithmetic op=ADD(w918, w915, w914, w913) -> (w917:u32)
              n425 = case shown="0, Default" w917 {
                tunnel: w951 -> [w961 _ _ _ _ _ _ _ _ _ _ _ _ _ _ _]
                tunnel: [w960 u32 1 ("Obs_state") u32 1 ("Obs_state") u32 1 ("Obs_state") u32 1 ("Obs_state") u32 1 ("Obs_state") u32 1 ("Obs_state") u32 1 ("Obs_state") u32 1 ("Obs_state") u32 1 ("Obs_state") u32 1 ("Obs_state") u32 1 ("Obs_state") u32 1 ("Obs_state") u32 1 ("Obs_state") u32 1 ("Obs_state") u32 1 ("Obs_state")] -> w950
                tunnel: ["" ("Error Msg") "ERROR: Lost channel 1 connection... - HandleObservationSync.vi state 251" ("Error Msg") "ERROR: Lost channel 2 connection...- HandleObservationSync.vi state 251" ("Error Msg") "ERROR: Lost channels 1 and 2 connection...- HandleObservationSync.vi state 251" ("Error Msg") "ERROR: Lost channel 3 connection...- HandleObservationSync.vi state 251" ("Error Msg") "ERROR: Lost channels 1 and  3 connection...- HandleObservationSync.vi state 251" ("Error Msg") "ERROR:  Lost channels 2 and  3 connection...- HandleObservationSync.vi state 251" ("Error Msg") "ERROR:  Lost channels 1, 2 and  3 connection...- HandleObservationSync.vi state 251" ("Error Msg") "ERROR: Lost channel 4 connection...- HandleObservationSync.vi state 251" ("Error Msg") "ERROR:  Lost channels 1 and 4 connection...- HandleObservationSync.vi state 251" ("Error Msg") "ERROR:  Lost channels 2 and 4 connection...- HandleObservationSync.vi state 251" ("Error Msg") "ERROR: Lost channels 1, 2 and 4 connection...- HandleObservationSync.vi state 251" ("Error Msg") "ERROR: Lost channels 3 and 4 connection...- HandleObservationSync.vi state 251" ("Error Msg") "ERROR: Lost channels 1, 3 and 4 connection...- HandleObservationSync.vi state 251" ("Error Msg") "ERROR: Lost channels 2, 3 and 4 connection...- HandleObservationSync.vi state 251" ("Error Msg") "ERROR: Lost channels 1, 2, 3 and 4 connection...- HandleObservationSync.vi state 251" ("Error Msg")] -> w916
                frame 0, Default {
                  n426 = Tick Count (ms)() -> (millisecond timer value=→"time307":u32)
                  n427 = Increment(x=w961) -> (x+1=w960:u32)
                }
                frame 1 {
                }
                frame 2 {
                }
                frame 3 {
                }
                frame 4 {
                }
                frame 5 {
                }
                frame 6 {
                }
                frame 7 {
                }
                frame 8 {
                }
                frame 9 {
                }
                frame 10 {
                }
                frame 11 {
                }
                frame 12 {
                }
                frame 13 {
                }
                frame 14 {
                }
                frame 15 {
                }
              }
            }
          }
          n428 = Bundle By Name(cluster=w883, "Obs_state"=w885, "cyclesDone"=u32 0, "Error Msg"=w880) -> (w887:refnum<class "S4GUI.lvclass">)
        }
        frame 252 {
          w1116 = 38 ("x")
          w1119 = 28 ("x")
          # "Se algum canal foi pra 38: Texp inválido \npara a configuração do CCD."
          # "Se algum canal foi pra 28: ERRO na inicialização."
          # "Espera terminar a execução da preparação\ndos 4 canais antes de ir ao proximo passo \nda Observação. E verifica se há pelo menos\n 1 canal habilitado."
          n429 = flat-sequence {
            tunnel: w1148 -> [w1293]
            tunnel: [w1293] -> w1147
            frame #0 {
              n430 = Tick Count (ms)() -> (millisecond timer value=→"time4":u32)
            }
          }
          n431 = call-dynamic "Read AcquisitionA.vi"("error in (no error)"=w1147, "S4ACS_GUI in"=w1157) -> ("error out"=w1145:errorcluster, "Acquisition.lvclass"=w1146:refnum<class "Acquisition.lvclass">, "S4ACS_GUI out"=w1159:refnum<class "S4GUI.lvclass">)  [unwired: 7 in]
          n432 = call "Read connection.vi"("error in (no error)"=w1145, "Server in"=w1146) -> ("error out"=w1143:errorcluster, "connection"=w1142:bool, "Server out"=w1144:refnum<class "Acquisition.lvclass">)  [unwired: 7 in]
          n433 = case shown="True" w1142 {
            tunnel: w1144 -> [w1276 w1292]
            tunnel: w1143 -> [w1275 w1291]
            tunnel: [w1276 w1289] -> w1160
            tunnel: [w1275 w1288] -> w1158
            tunnel: [0 ("State") w1278] -> w1115
            frame False {
            }
            frame True {
              n434 = call-dynamic "Read Channel.vi"("error in (no error)"=w1291, "Acquisition in"=w1292) -> ("error out"=w1287:errorcluster, "Channel.lvclass"=w1286:refnum<class "Channel.lvclass">, "Acquisition out"=w1290:refnum<class "Acquisition.lvclass">)  [unwired: 7 in]
              n435 = call-dynamic "Read State Machine.vi"("error in (no error)"=w1287, "Device in"=w1286) -> ("error out"=w1280:errorcluster, "State Machine.lvclass"=w1282:refnum<class "State Machine.lvclass">, "Device out"=w1284:refnum<class "Channel.lvclass">)  [unwired: 7 in]
              n436 = call-dynamic "Read State.vi"("error in (no error)"=w1280, "State Machine in"=w1282) -> ("error out"=w1279:errorcluster, "State"=w1278:i32, "State Machine out"=w1281:refnum<class "State Machine.lvclass">)  [unwired: 7 in]
              n437 = call-dynamic "Write State Machine.vi"("error in (no error)"=w1279, "State Machine.lvclass"=w1281, "Device in"=w1284) -> ("error out"=w1283:errorcluster, "Device out"=w1285:refnum<class "Channel.lvclass">)  [unwired: 7 in]
              n438 = call-dynamic "Write Channel.vi"("error in (no error)"=w1283, "Channel.lvclass"=w1285, "Acquisition in"=w1290) -> ("error out"=w1288:errorcluster, "Acquisition out"=w1289:refnum<class "Acquisition.lvclass">)  [unwired: 7 in]
            }
          }
          n439 = call-dynamic "Write AcquisitionA.vi"("error in (no error)"=w1158, "Acquisition.lvclass"=w1160, "S4ACS_GUI in"=w1159) -> ("error out"=w1154:errorcluster, "S4ACS_GUI out"=w1153:refnum<class "S4GUI.lvclass">)  [unwired: 7 in]
          n440 = call "Read AcquisitionB.vi"("error in (no error)"=w1154, "S4ACS_GUI in"=w1153) -> ("error out"=w1137:errorcluster, "Acquisition.lvclass"=w1140:refnum<class "Acquisition.lvclass">, "S4ACS_GUI out"=w1141:refnum<class "S4GUI.lvclass">)  [unwired: 7 in]
          n441 = call "Read connection.vi"("error in (no error)"=w1137, "Server in"=w1140) -> ("error out"=w1136:errorcluster, "connection"=w1138:bool, "Server out"=w1139:refnum<class "Acquisition.lvclass">)  [unwired: 7 in]
          n442 = case shown="True" w1138 {
            tunnel: w1139 -> [w1258 w1274]
            tunnel: w1136 -> [w1257 w1273]
            tunnel: [w1258 w1271] -> w1135
            tunnel: [w1257 w1270] -> w1134
            tunnel: [0 ("State") w1260] -> w1114
            frame False {
            }
            frame True {
              n443 = call-dynamic "Read Channel.vi"("error in (no error)"=w1273, "Acquisition in"=w1274) -> ("error out"=w1269:errorcluster, "Channel.lvclass"=w1268:refnum<class "Channel.lvclass">, "Acquisition out"=w1272:refnum<class "Acquisition.lvclass">)  [unwired: 7 in]
              n444 = call-dynamic "Read State Machine.vi"("error in (no error)"=w1269, "Device in"=w1268) -> ("error out"=w1262:errorcluster, "State Machine.lvclass"=w1264:refnum<class "State Machine.lvclass">, "Device out"=w1266:refnum<class "Channel.lvclass">)  [unwired: 7 in]
              n445 = call-dynamic "Read State.vi"("error in (no error)"=w1262, "State Machine in"=w1264) -> ("error out"=w1261:errorcluster, "State"=w1260:i32, "State Machine out"=w1263:refnum<class "State Machine.lvclass">)  [unwired: 7 in]
              n446 = call-dynamic "Write State Machine.vi"("error in (no error)"=w1261, "State Machine.lvclass"=w1263, "Device in"=w1266) -> ("error out"=w1265:errorcluster, "Device out"=w1267:refnum<class "Channel.lvclass">)  [unwired: 7 in]
              n447 = call-dynamic "Write Channel.vi"("error in (no error)"=w1265, "Channel.lvclass"=w1267, "Acquisition in"=w1272) -> ("error out"=w1270:errorcluster, "Acquisition out"=w1271:refnum<class "Acquisition.lvclass">)  [unwired: 7 in]
            }
          }
          n448 = call "Write AcquisitionB.vi"("error in (no error)"=w1134, "Acquisition.lvclass"=w1135, "S4ACS_GUI in"=w1141) -> ("error out"=w1152:errorcluster, "S4ACS_GUI out"=w1151:refnum<class "S4GUI.lvclass">)  [unwired: 7 in]
          n449 = call-dynamic "Read AcquisitionC.vi"("error in (no error)"=w1152, "S4ACS_GUI in"=w1151) -> ("error out"=w1132:errorcluster, "Acquisition.lvclass"=w1133:refnum<class "Acquisition.lvclass">, "S4ACS_GUI out"=w1156:refnum<class "S4GUI.lvclass">)  [unwired: 7 in]
          n450 = call "Read connection.vi"("error in (no error)"=w1132, "Server in"=w1133) -> ("error out"=w1131:errorcluster, "connection"=w1129:bool, "Server out"=w1130:refnum<class "Acquisition.lvclass">)  [unwired: 7 in]
          n451 = case shown="True" w1129 {
            tunnel: w1130 -> [w1240 w1256]
            tunnel: w1131 -> [w1239 w1255]
            tunnel: [w1240 w1253] -> w1128
            tunnel: [w1239 w1252] -> w1127
            tunnel: [0 ("State") w1242] -> w1113
            frame False {
            }
            frame True {
              n452 = call-dynamic "Read Channel.vi"("error in (no error)"=w1255, "Acquisition in"=w1256) -> ("error out"=w1251:errorcluster, "Channel.lvclass"=w1250:refnum<class "Channel.lvclass">, "Acquisition out"=w1254:refnum<class "Acquisition.lvclass">)  [unwired: 7 in]
              n453 = call-dynamic "Read State Machine.vi"("error in (no error)"=w1251, "Device in"=w1250) -> ("error out"=w1244:errorcluster, "State Machine.lvclass"=w1246:refnum<class "State Machine.lvclass">, "Device out"=w1248:refnum<class "Channel.lvclass">)  [unwired: 7 in]
              n454 = call-dynamic "Read State.vi"("error in (no error)"=w1244, "State Machine in"=w1246) -> ("error out"=w1243:errorcluster, "State"=w1242:i32, "State Machine out"=w1245:refnum<class "State Machine.lvclass">)  [unwired: 7 in]
              n455 = call-dynamic "Write State Machine.vi"("error in (no error)"=w1243, "State Machine.lvclass"=w1245, "Device in"=w1248) -> ("error out"=w1247:errorcluster, "Device out"=w1249:refnum<class "Channel.lvclass">)  [unwired: 7 in]
              n456 = call-dynamic "Write Channel.vi"("error in (no error)"=w1247, "Channel.lvclass"=w1249, "Acquisition in"=w1254) -> ("error out"=w1252:errorcluster, "Acquisition out"=w1253:refnum<class "Acquisition.lvclass">)  [unwired: 7 in]
            }
          }
          n457 = call-dynamic "Write AcquisitionC.vi"("error in (no error)"=w1127, "Acquisition.lvclass"=w1128, "S4ACS_GUI in"=w1156) -> ("error out"=w1150:errorcluster, "S4ACS_GUI out"=w1149:refnum<class "S4GUI.lvclass">)  [unwired: 7 in]
          n458 = call-dynamic "Read AcquisitionD.vi"("error in (no error)"=w1150, "S4ACS_GUI in"=w1149) -> ("error out"=w1124:errorcluster, "Acquisition.lvclass"=w1126:refnum<class "Acquisition.lvclass">, "S4ACS_GUI out"=w1155:refnum<class "S4GUI.lvclass">)  [unwired: 7 in]
          n459 = call "Read connection.vi"("error in (no error)"=w1124, "Server in"=w1126) -> ("error out"=w1123:errorcluster, "connection"=w1122:bool, "Server out"=w1125:refnum<class "Acquisition.lvclass">)  [unwired: 7 in]
          n460 = case shown="True" w1122 {
            tunnel: w1125 -> [w1222 w1238]
            tunnel: w1123 -> [w1221 w1237]
            tunnel: [w1222 w1235] -> w1121
            tunnel: [w1221 w1234] -> w1120
            tunnel: [0 ("State") w1224] -> w1112
            frame False {
            }
            frame True {
              n461 = call-dynamic "Read Channel.vi"("error in (no error)"=w1237, "Acquisition in"=w1238) -> ("error out"=w1233:errorcluster, "Channel.lvclass"=w1232:refnum<class "Channel.lvclass">, "Acquisition out"=w1236:refnum<class "Acquisition.lvclass">)  [unwired: 7 in]
              n462 = call-dynamic "Read State Machine.vi"("error in (no error)"=w1233, "Device in"=w1232) -> ("error out"=w1226:errorcluster, "State Machine.lvclass"=w1228:refnum<class "State Machine.lvclass">, "Device out"=w1230:refnum<class "Channel.lvclass">)  [unwired: 7 in]
              n463 = call-dynamic "Read State.vi"("error in (no error)"=w1226, "State Machine in"=w1228) -> ("error out"=w1225:errorcluster, "State"=w1224:i32, "State Machine out"=w1227:refnum<class "State Machine.lvclass">)  [unwired: 7 in]
              n464 = call-dynamic "Write State Machine.vi"("error in (no error)"=w1225, "State Machine.lvclass"=w1227, "Device in"=w1230) -> ("error out"=w1229:errorcluster, "Device out"=w1231:refnum<class "Channel.lvclass">)  [unwired: 7 in]
              n465 = call-dynamic "Write Channel.vi"("error in (no error)"=w1229, "Channel.lvclass"=w1231, "Acquisition in"=w1236) -> ("error out"=w1234:errorcluster, "Acquisition out"=w1235:refnum<class "Acquisition.lvclass">)  [unwired: 7 in]
            }
          }
          n466 = call-dynamic "Write AcquisitionD.vi"("error in (no error)"=w1120, "Acquisition.lvclass"=w1121, "S4ACS_GUI in"=w1155) -> ("error out"=w1106:errorcluster, "S4ACS_GUI out"=w1107:refnum<class "S4GUI.lvclass">)  [unwired: 7 in]
          n467 = Equal?(x=w1116, y=w1115) -> (x = y?=w1102:bool)
          n468 = Equal?(x=w1119, y=w1115) -> (x = y?=w1097:bool)
          n469 = Equal?(x=w1116, y=w1114) -> (x = y?=w1096:bool)
          n470 = Equal?(x=w1119, y=w1114) -> (x = y?=w1098:bool)
          n471 = Equal?(x=w1116, y=w1113) -> (x = y?=w1095:bool)
          n472 = Equal?(x=w1119, y=w1113) -> (x = y?=w1099:bool)
          n473 = Equal?(x=w1116, y=w1112) -> (x = y?=w1101:bool)
          n474 = Equal?(x=w1119, y=w1112) -> (x = y?=w1100:bool)
          n475 = call-dynamic "VerifyAcqIdle.vi"("error in (no error)"=w1106, "S4GUI in"=w1107) -> ("error out"=w1104:errorcluster, "all disabled"=w1094:bool, "idle"=w1103:bool, "S4GUI out"=w1105:refnum<class "S4GUI.lvclass">)  [unwired: 6 in]
          n476 = Compound Arithmetic op=OR(w1097, w1098, w1099, w1100) -> (w1111:bool)
          n477 = Compound Arithmetic op=OR(w1102, w1096, w1095, w1101) -> (w1110:bool)
          n478 = Build Array(w1111, w1110) -> (w1109:bool[])
          n479 = Boolean Array To Number(Boolean array=w1109) -> (number=w1108:u32)
          n480 = case shown="0, Default" w1108 {
            tunnel: w1105 -> [w1171 w1203 w1216 w1220]
            tunnel: [w1170 w1202 w1215 w1219] -> w1117
            tunnel: w1118 -> [w1172 _ _ _]
            tunnel: w1103 -> [w1168 _ _ _]
            tunnel: w1102 -> [_ _ w1213 _]
            tunnel: w1096 -> [_ _ w1212 _]
            tunnel: w1095 -> [_ _ w1211 _]
            tunnel: w1101 -> [_ _ w1210 _]
            tunnel: w1100 -> [_ w1195 _ _]
            tunnel: w1099 -> [_ w1196 _ _]
            tunnel: w1098 -> [_ w1197 _ _]
            tunnel: w1097 -> [_ w1198 _ _]
            tunnel: w1094 -> [w1161 _ _ _]
            frame 0, Default {
              n481 = local read "time307"() -> (w1166:u32)
              n482 = Tick Count (ms)() -> (millisecond timer value=w1167:u32)
              n483 = Subtract(x=w1167, y=w1166) -> (x-y=w1165:u32)
              n484 = Greater?(x=w1165, y=u32 10000) -> (0:w1163:bool)
              n485 = case shown="False" w1163 {
                tunnel: w1172 -> [w1177 _]
                tunnel: [w1176 u32 1 ("Obs_state")] -> w1169
                tunnel: w1168 -> [w1175 _]
                tunnel: [w1174 w1188] -> w1162
                tunnel: w1161 -> [w1173 _]
                frame False {
                  n486 = case shown="True" w1173 {
                    tunnel: w1177 -> [w1181 _]
                    tunnel: [w1180 u32 1 ("Obs_state")] -> w1176
                    tunnel: w1175 -> [w1179 _]
                    tunnel: ["" "ERROR: No channel enabled."] -> w1174
                    frame False {
                      # "At least 1 channel enabled."
                      n487 = disable-structure shown="Enabled" {
                        disable-tunnel: [299 ("t") 300] -> w1182
                        frame Disabled {
                        }
                        frame Enabled {
                        }
                      }
                      n488 = Select(t=w1182, s=w1179, f=w1181) -> (s? t:f=w1180:u32)
                    }
                    frame True {
                      # "No channel enabled"
                    }
                  }
